vi "Difference.vi"(10 "Angle":dbl, 11 "Gyro":dbl) -> (3 "Difference":dbl)   [LabVIEW 2020]
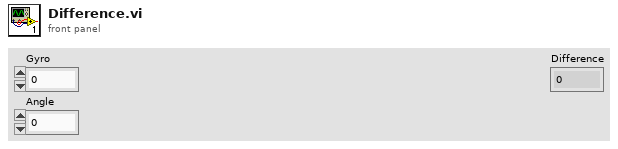
[diagram p1: front panel]
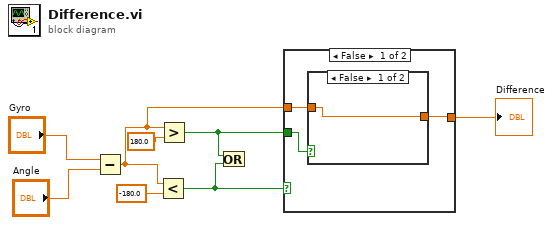
[diagram p0: block diagram]
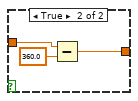
[diagram p2: hidden frame]
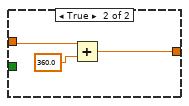
[diagram p3: hidden frame]
diagram:
  n1 = Subtract(x="Gyro", y="Angle") -> (x-y=w2:dbl)
  n2 = Less?(x=w2, y=-180.0) -> (x < y?=w4:bool)
  n3 = Greater?(x=w2, y=180.0) -> (0:w3:bool)
  n4 = Or(x=w3, y=w4) -> ()  [unwired: 1 out]
  n5 = case shown="False" w4 {
    tunnel: w3 -> [w11 _]
    tunnel: w2 -> [w10 w18]
    tunnel: [w9 w16] -> w1
    frame False {
      n6 = case shown="False" w11 {
        tunnel: w10 -> [w12 w14]
        tunnel: [w12 w13] -> w9
        frame False {
        }
        frame True {
          n7 = Subtract(x=w14, y=360.0) -> (x-y=w13:dbl)
        }
      }
    }
    frame True {
      n8 = Add(x=w18, y=360.0) -> (x+y=w16:dbl)
    }
  }
  "Difference" <- w1
